vi "Get Scaling Coefficients.vi"(0 "device session in":refnum<class "Device Session.lvclass">, 11 "error in":errorcluster) -> (4 "device session out":refnum<class "Device Session.lvclass">, 6 "scaling coefficients":cluster{"gain":dbl, "offset":dbl}[](array[cluster]), 15 "error out":errorcluster)   [LabVIEW 2015, in "Device Session.lvclass"]
doc: "Returns the gain and offset values that you can use to scale data. This VI returns the scaling coefficients for each channel specified in the <B>channels to stream</B> parameter of the <B>Configure Acquisition</B> VI. You must run the <B>Configure Acquisition</B> VI before running this VI.\n\n<B>Input Parameters</B>\n\n<B>device session in</B> is a reference to the session containing sessions to all instrument design libraries used in this sample project. This parameter is obtained from the 'Open Session' VI.\n\n<B>error in</B> describes error conditions that occur before this node runs. This input provides standard 'error in' functionality.\n\n<B>Output Parameters</B>\n\n<B>device session out</B> passes a reference to the session to the next VI.\n\n<B>scaling coefficients</B> contains the scaling coefficients.\n\n<B>scaling coefficients.gain</B> is the gain coefficient.\n\n<B>scaling coefficients.offset</B> is the offset coefficient.\n\n<B>error out</B> contains error information. This output provides standard 'error out' functionality."
uses:
  Device Session.lvclass
  Device Session.lvclass/Device Session.ctl
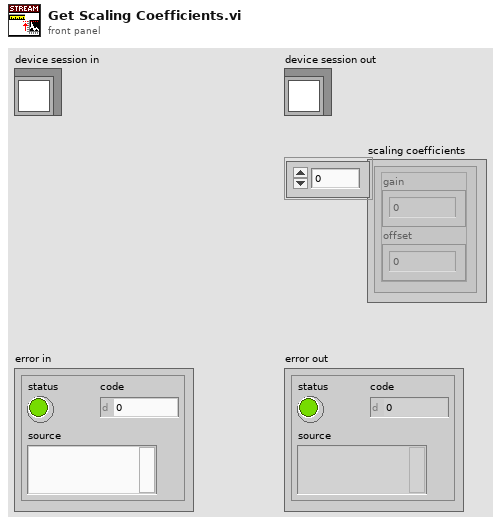
[diagram p1: front panel]
types:
  T1 = typedef "Device Session.lvclass/Device Session Object.ctl" = cluster{"ni5171R FPGA Reference":T2, "niHSAI config":refnum<class "niHSAI Config v1 Host.lvclass">, "configured scaling coefficients":cluster{"gain":dbl, "offset":dbl}[], "number of channels to stream":u8, "selected acq channels":bool[], "number of channels":u32, "actual channel configuration":T3[], "configured channels":bool[], "sample clock rate (Hz)":dbl}
  T2 = typedef "Device Session.lvclass/FPGA Refnum.ctl" = refnum<k20>
  T3 = typedef "niHSAI Types v1 Host.lvlib/Channel Configuration.ctl" = cluster{"channel":u32, "coupling":T4, "impedance":T5, "bandwidth":T6, "vertical range":dbl, "vertical offset":dbl}
  T4 = typedef "niHSAI Types v1 Host.lvlib/Coupling.ctl" = enum8{"Default", "DC", "AC"}
  T5 = typedef "niHSAI Types v1 Host.lvlib/Impedance.ctl" = enum8{"Default", "1 mega ohm", "50 ohm"}
  T6 = typedef "niHSAI Types v1 Host.lvlib/Bandwidth.ctl" = enum8{"Default", "Full Bandwidth", "Anti-alias Filter"}
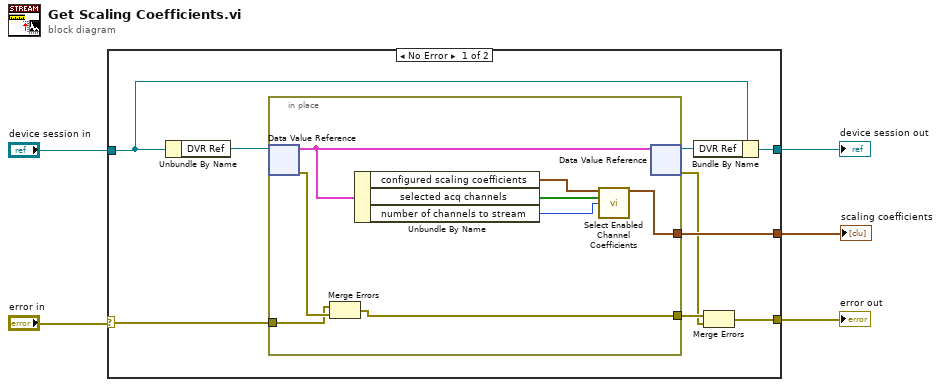
[diagram p0: block diagram]
diagram:
  n1 = case shown="No Error" "error in" {
    selector: "error in" -> [w14 w24]
    tunnel: [w9 w24] -> w4
    tunnel: "device session in" -> [w12 w23]
    tunnel: [w10 w23] -> w2
    tunnel: [w7 _] -> w1
    frame No Error {
      n2 = Unbundle By Name(w12) -> ("DVR Ref"=w13:refnum<data-value>)
      n3 = in-place {
        in-place-border: w14 -> [w21]
        in-place-border: [w19] -> w8
        in-place-border: [w17] -> w7
        n4 = in-place-dvr #1(w13) -> (w20:T1, w22:errorcluster)
        n5 = Merge Errors(w21, w22) -> (w19:errorcluster)
        n6 = Unbundle By Name(w20) -> ("configured scaling coefficients"=w18:cluster{"gain":dbl, "offset":dbl}[], "selected acq channels"=w16:bool[], "number of channels to stream"=w15:u8)
        n7 = call "Select Enabled Channel Coefficients.vi"("configured scaling coefficients"=w18, "selected acq channels to stream"=w16, "number of selected acq channels to stream"=w15) -> ("streamed scaling coefficients"=w17:cluster{"gain":dbl, "offset":dbl}[])  [unwired: 12 in]
        n8 = in-place-dvr #1(w20) -> (w11:refnum<data-value>, w6:errorcluster)
      }
      n9 = Bundle By Name(cluster=w12, "DVR Ref"=w11) -> (w10:refnum<class "Device Session.lvclass">)
      n10 = Merge Errors(w8, w6) -> (w9:errorcluster)
    }
    frame Error {
    }
  }
  "error out" <- w4
  "device session out" <- w2
  "scaling coefficients" <- w1
